vi "Shift Registers.vi"() -> ()   [LabVIEW 2015]
panel:
  out "Final Value (For)":dbl
  out "Final Value (While)":dbl
  in  "stop":bool
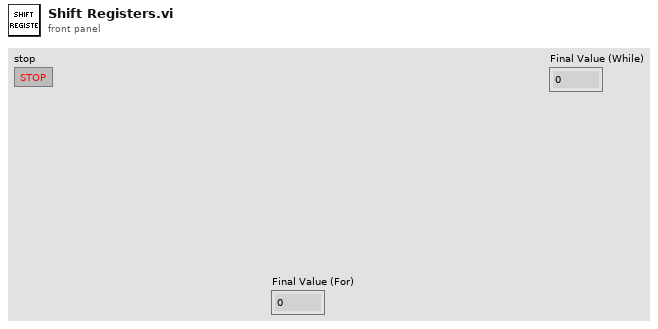
[diagram p1: front panel]
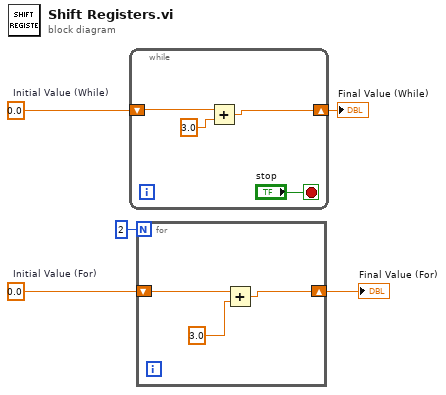
[diagram p0: block diagram]
diagram:
  w3 = 0.0  # Initial Value (For)
  w5 = 0.0  # Initial Value (While)
  n1 = while {
    shift-right: [w7] -> w4
    shift-left: w5 -> [w9]
    stop <- "stop" stop-if-true
    n2 = Add(x=w9, y=3.0) -> (x+y=w7:dbl)
  }
  "Final Value (While)" <- w4
  n3 = for {
    N: 2 -> [_]
    shift-right: [w10] -> w2
    shift-left: w3 -> [w11]
    n4 = Add(x=w11, y=3.0) -> (x+y=w10:dbl)
  }
  "Final Value (For)" <- w2
